vi "Read ID.vi"(8 "error in (no error)":errorcluster, 11 "189 in":refnum<class "189.lvclass">) -> (0 "error out":errorcluster, 3 "189 out":refnum<class "189.lvclass">)   [LabVIEW 2015, in "189.lvclass"]
doc: "VI used to Read Hardware ID"
uses:
  189.lvclass
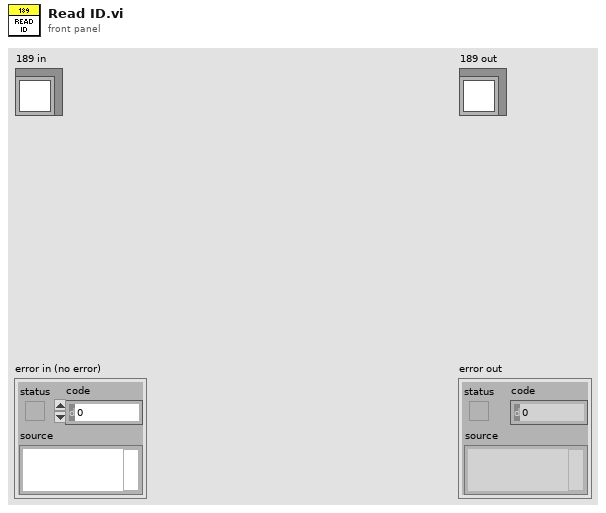
[diagram p1: front panel]
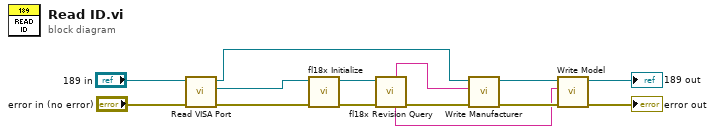
[diagram p0: block diagram]
diagram:
  n1 = call-dynamic "Read VISA Port.vi"("error in (no error)"="error in (no error)", "Device in"="189 in") -> ("error out"=w12:errorcluster, "VISA Port"=w13:refnum<visa-resource-name>, "Device out"=w5:refnum<class "189.lvclass">)  [unwired: 7 in]
  n2 = call <instrlib>:"fl18x Initialize.vi"("error in (no error)"=w12, "VISA resource name"=w13) -> ("error out"=w14:errorcluster, "VISA resource name out"=w9:refnum<visa-resource-name>)  [unwired: 8 in]
  n3 = call <instrlib>:"fl18x Revision Query.vi"("error in (no error)"=w14, "VISA session"=w9) -> ("error out"=w8:errorcluster, "Modelo"=w2:string, "Fabricante"=w4:string)  [unwired: 4 in, 3 out]
  n4 = call-dynamic "Write Manufacturer.vi"("error in (no error)"=w8, "Manufacturer"=w4, "Device in"=w5) -> ("error out"=w7:errorcluster, "Device out"=w3:refnum<class "189.lvclass">)  [unwired: 7 in]
  n5 = call-dynamic "Write Model.vi"("error in (no error)"=w7, "Model"=w2, "Device in"=w3) -> ("error out"=→"error out":errorcluster, "Device out"=→"189 out":refnum<class "189.lvclass">)  [unwired: 7 in]
